vi "for loop count.vi"() -> ()   [LabVIEW 2016]
panel:
  out "For Loop Count":i32(graph)
  in  "Number of Iterations":i32
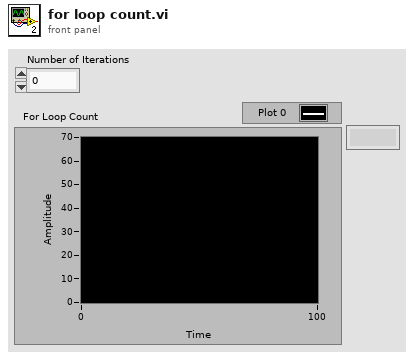
[diagram p1: front panel]
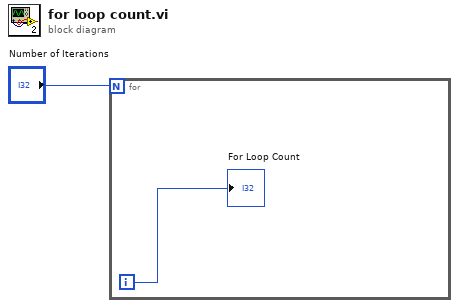
[diagram p0: block diagram]
diagram:
  n1 = for {
    N: "Number of Iterations" -> [_]
    i -> [w2]
    "For Loop Count" <- w2
  }
